vi "SG Configure.vi"(11 "Semiconductor Module Context":T1) -> (0 "error out":errorcluster)   [LabVIEW 2014]
uses:
  <vilib>/NI_TestStand_SemiconductorModule/NI_TestStand_Semiconductor_Module.lvlibp/PinMap/General/SemiconductorModuleContext.ctl
  <vilib>/NI_TestStand_SemiconductorModule/NI_TestStand_Semiconductor_Module.lvlibp
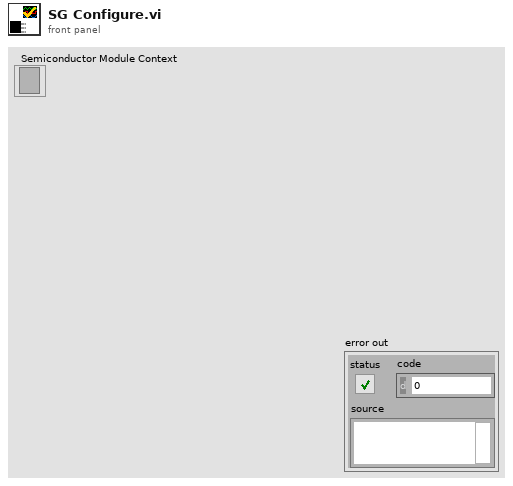
[diagram p1: front panel]
types:
  T1 = typedef "NI_TestStand_Semiconductor_Module.lvlibp/SemiconductorModuleContext.ctl" = refnum<k7>
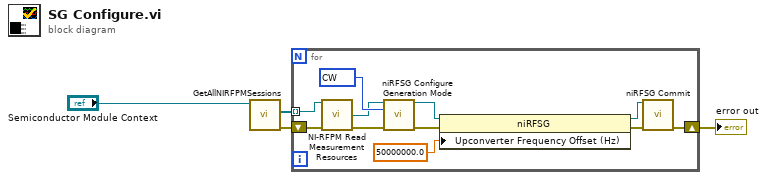
[diagram p0: block diagram]
diagram:
  n1 = call <vilib>:"GetAllNIRFPMSessions.vi"("Semiconductor Module Context"="Semiconductor Module Context") -> ("error out"=w4:errorcluster, "Instrument Sessions"=w2:refnum<k15>[])  [unwired: 8 in, 1 out]
  n2 = for {
    shift-right: [w7] -> w1
    shift-left: w4 -> [w14]
    tunnel: w2 -> [w15] mode=indexing
    w10 = 1000 items=["CW"=1000, "Arb Waveform"=1001, "Script"=1002] ("generation mode")
    n3 = call <instrlib>:"NI-RFPM Read Measurement Resources.vi"("NI-5530 handle in"=w15, "error in"=w14) -> ("RFSG handle"=w6:refnum<k15>, "error out"=w5:errorcluster)  [unwired: 9 in, 3 out]
    n4 = call <instrlib>:"niRFSG Configure Generation Mode.vi"("instrument handle"=w6, "generation mode"=w10, "error in"=w5) -> ("instrument handle out"=w11:refnum<k15>, "error out"=w13:errorcluster)  [unwired: 11 in]
    n5 = property class="niRFSG"(reference=w11, error in=w13, "Upconverter Frequency Offset (Hz)"=50000000.0 ("Device Specific:Vector Signal Transceiver:Upconverter:Frequency Offset (Hz)")) -> (reference out=w9:refnum<k15>, error out=w8:errorcluster)
    n6 = call <instrlib>:"niRFSG Commit.vi"("instrument handle"=w9, "error in"=w8) -> ("error out"=w7:errorcluster)  [unwired: 12 in, 1 out]
  }
  "error out" <- w1
